vi "findMag_2.vi"(2 "error in (no error)":errorcluster, 3 "voltages":dbl[](array[numeric]), 4 "sens":dbl=0.15, 5 "times":dbl[](array[numeric])) -> (0 "error out":errorcluster, 1 "magfound":dbl)   [LabVIEW 2016]
panel:
  in  "num":dbl=5.0
  out "npeak":dbl
  out "ppeak":dbl
  in  "freq":dbl=1367000.0
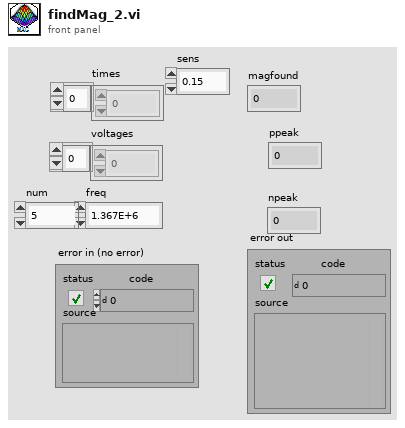
[diagram p1: front panel]
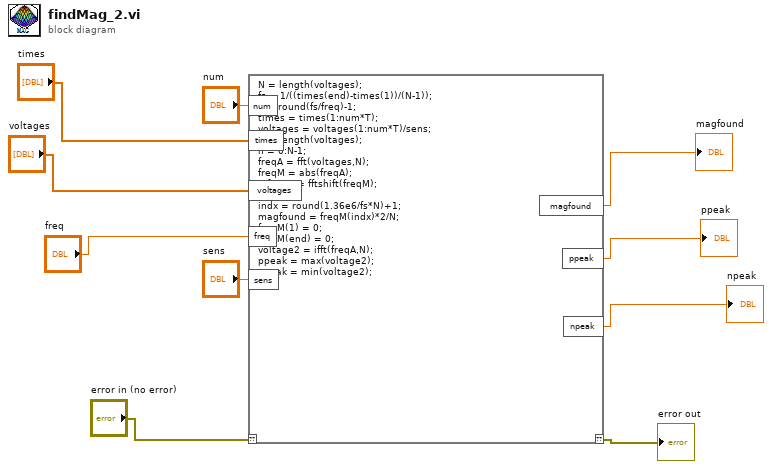
[diagram p0: block diagram]
diagram:
  n1 = script code="N = length(voltages);\nfs = 1/((times(end)-times(1))/(N-1));\nT = round(fs/freq)-1;\ntimes = times(1:num*T);\nvoltages = voltages(1:num*T)/sens;\nN = length(voltages);\nn = 0:N-1;\nfreqA = fft(voltages,N);\nfreqM = abs(freqA);\n%freqM = fftshift(freqM);\nf=n*fs/N;\nindx = round(1.36e6/fs*N)+1;\nmagfound = freqM(indx)*2/N;\nfreqM(1) = 0;\nfreqM(end) = 0;\nvoltage2 = ifft(freqA,N);\nppeak = max(voltage2);\nnpeak = min(voltage2);"("??"="error in (no error)", "times"="times", "voltages"="voltages", "freq"="freq", "num"="num", "sens"="sens") -> ("??"=→"error out":errorcluster, "magfound"=→"magfound":dbl, "ppeak"=→"ppeak":dbl, "npeak"=→"npeak":dbl)
